vi "EditOptions.vi"(8 "error in":errorcluster, 11 "Submodule EOL":refnum<class "Submodule EOL.lvclass">) -> (0 "error out":errorcluster, 1 "edit options":T1, 2 "subnodes class":T2, 3 "Submodule EOL out":refnum<class "Submodule EOL.lvclass">)   [LabVIEW 2025, in "Submodule EOL.lvlib" / "Submodule EOL.lvclass"]
doc: "Contains the options for the Menu that will be displayed when doing right click on an item.\nThe sub nodes class configures which nodes can be added to this nodes\nAnd the edit options determine which options are available for the node.\nThis configuration is stored in this VI in case some dynamic configuration is required for the menu options or sub nodes.\nCopyright 2017 National Instruments Corporation\n\nLicensed under the Apache License, Version 2.0 (the \"License\"); you may not use this file except in compliance with the License. You may obtain a copy of the License at http://www.apache.org/licenses/LICENSE-2.0\nUnless required by applicable law or agreed to in writing, software distributed under the License is distributed on an \"AS IS\" BASIS, WITHOUT WARRANTIES OR CONDITIONS OF ANY KIND, either express or implied. See the License for the specific language governing permissions and limitations under the License."
uses:
  Submodule EOL.lvclass
  Users/Public/Documents/Sandia National Labs/TSS Plugin/CEF.lvlibp/Node/NodeMenuOptions.ctl
  Users/Public/Documents/Sandia National Labs/TSS Plugin/CEF.lvlibp/Node/SubNodeCluster.ctl
  Submodule EOL.lvclass/Submodule EOL.ctl
  Users/Public/Documents/Sandia National Labs/TSS Plugin/CEF.lvlibp/Node/CEF_Node.lvclass
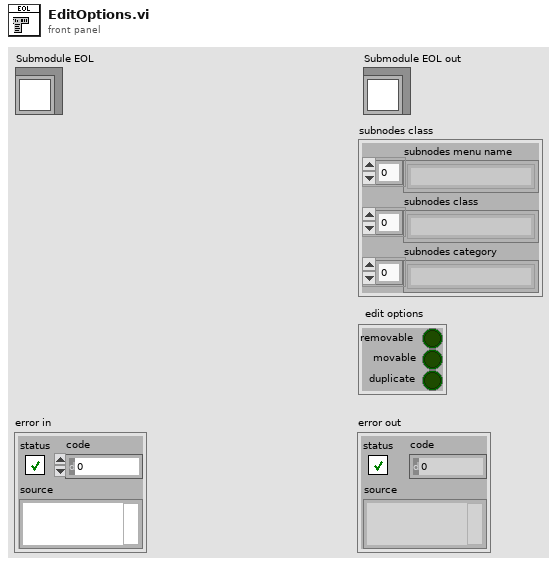
[diagram p1: front panel]
types:
  T1 = cluster{"removable":bool, "movable":bool, "duplicate":bool}
  T2 = cluster{"subnodes menu name":string[], "subnodes class":string[], "subnodes category":string[]}
  T3 = typedef "CEF.lvlibp/CEF_Node.lvclass/SubNodeCluster.ctl" = cluster{"subnodes menu name":string[], "subnodes class":string[], "subnodes category":string[]}
  T4 = typedef "CEF.lvlibp/CEF_Node.lvclass/NodeMenuOptions.ctl" = cluster{"removable":bool, "movable":bool, "duplicate":bool}
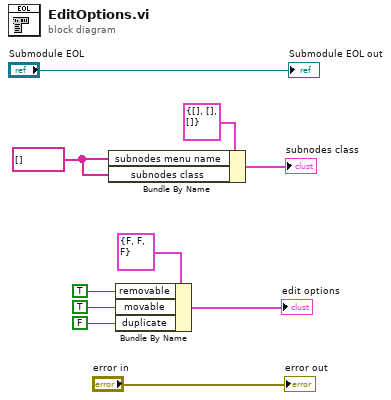
[diagram p0: block diagram]
diagram:
  w4 = string[] [] ("subnodes menu name")
  n1 = Bundle By Name(cluster=T3 {"subnodes menu name"=[], "subnodes class"=[], "subnodes category"=[]} ("subnodes class"), "subnodes menu name"=w4, "subnodes class"=w4) -> (→"subnodes class":T3)
  n2 = Bundle By Name(cluster=T4 {"removable"=FALSE, "movable"=FALSE, "duplicate"=FALSE} ("edit options"), "removable"=TRUE ("Removable"), "movable"=TRUE ("Movable"), "duplicate"=FALSE ("Duplicate")) -> (→"edit options":T4)
  "error out" <- "error in"
  "Submodule EOL out" <- "Submodule EOL"
